vi "Euler 004.vi"() -> ()   [LabVIEW 2021]
panel:
  out "largest palindrome":i32
  out "sorted array":i32[](array[numeric])
  out "max value":i32
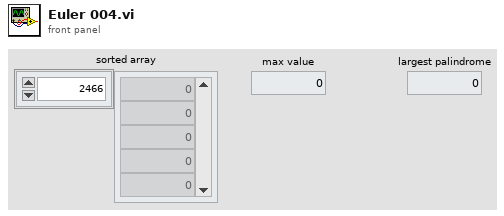
[diagram p1: front panel]
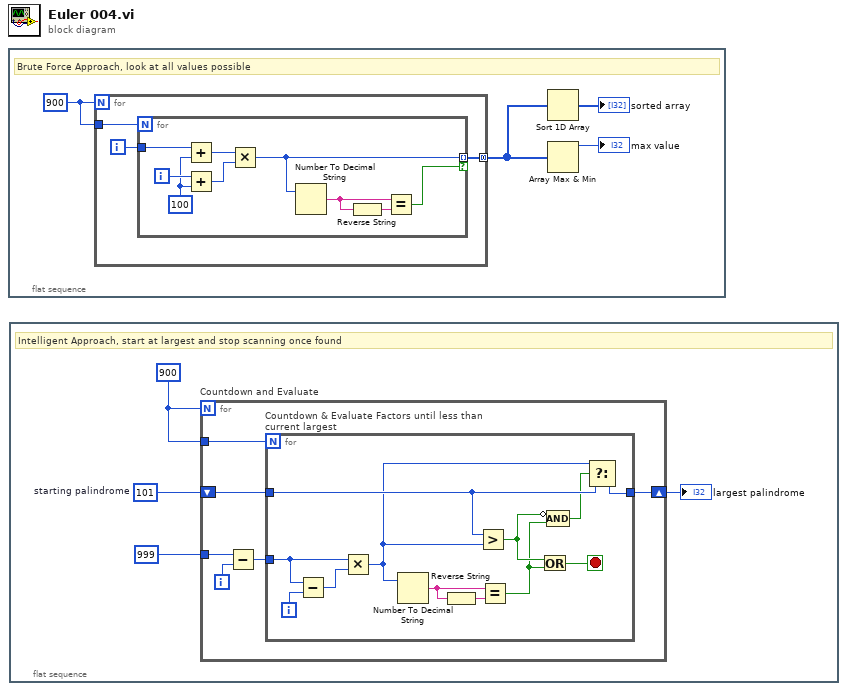
[diagram p0: block diagram]
diagram:
  n1 = flat-sequence {
    frame #0 {
      w4 = 900
      # "Brute Force Approach, look at all values possible"
      n2 = for {
        N: w4 -> [_]
        tunnel: w4 -> [w6]
        tunnel: [w5] -> w2 mode=concatenating
        i -> [w7]
        n3 = for {
          N: w6 -> [_]
          tunnel: w7 -> [w16]
          tunnel: [w15] -> w5 mode=indexing if=w14
          i -> [w11]
          w8 = 100 ("y")
          n4 = Add(x=w16, y=w8) -> (x+y=w9:i32)
          n5 = Add(x=w11, y=w8) -> (x+y=w10:i32)
          n6 = Multiply(x=w9, y=w10) -> (x*y=w15:i32)
          n7 = Number To Decimal String(number=w15) -> (decimal integer string=w12:string)  [unwired: 1 in]
          n8 = Reverse String(1:w12) -> (0:w13:string)
          n9 = Equal?(x=w12, y=w13) -> (x = y?=w14:bool)
        }
      }
      n10 = Sort 1D Array(array=w2) -> (sorted array=→"sorted array":i32[])
      n11 = Array Max & Min(array=w2) -> (max value=→"max value":i32)  [unwired: 3 out]
    }
  }
  n12 = flat-sequence {
    frame #0 {
      w19 = 101  # starting palindrome
      w17 = 900
      # "Intelligent Approach, start at largest and stop scanning once found"
      n13 = for "Countdown and Evaluate" {
        N: w17 -> [_]
        tunnel: 999 ("y") -> [w24]
        shift-right: [w22] -> w18
        shift-left: w19 -> [w23]
        tunnel: w17 -> [w21]
        i -> [w25]
        n14 = Subtract(x=w24, y=w25) -> (x-y=w26:i32)
        n15 = for "Countdown & Evaluate Factors until less than current largest" {
          N: w21 -> [_]
          tunnel: w26 -> [w32]
          tunnel: w23 -> [w34]
          tunnel: [w33] -> w22
          i -> [w38]
          stop <- w31 stop-if-true
          n16 = Subtract(x=w32, y=w38) -> (x-y=w37:i32)
          n17 = Multiply(x=w32, y=w37) -> (x*y=w30:i32)
          n18 = Number To Decimal String(number=w30) -> (decimal integer string=w36:string)  [unwired: 1 in]
          n19 = Reverse String(1:w36) -> (0:w35:string)
          n20 = Greater?(x=w34, y=w30) -> (0:w29:bool)
          n21 = Equal?(x=w36, y=w35) -> (x = y?=w27:bool)
          n22 = Or(x=w29, y=w27) -> (x .or. y?=w31:bool)
          n23 = Compound Arithmetic op=AND(invert w29, w27) -> (w28:bool)
          n24 = Select(t=w30, s=w28, f=w34) -> (s? t:f=w33:i32)
        }
      }
      "largest palindrome" <- w18
    }
  }
